vi "InitializeSlowDAQ.vi"(11 "Negative Channels in":i32[](array[numeric])=[3, 5, 7, 9, 199, 199, 199, 199, 199, 199, 199]) -> (0 "error out":errorcluster, 1 "Handle Out":i32, 2 "IO Types Out":string[](array[string]), 3 "Positive Channels 2":i32[](array[numeric])=[2, 4, 6, 8, 0, 1, 10, 11, 12, 13, 14], 5 "Negative Channels out":i32[](array[numeric])=[3, 5, 7, 9, 199, 199, 199, 199, 199, 199, 199])   [LabVIEW 2022 SP3]
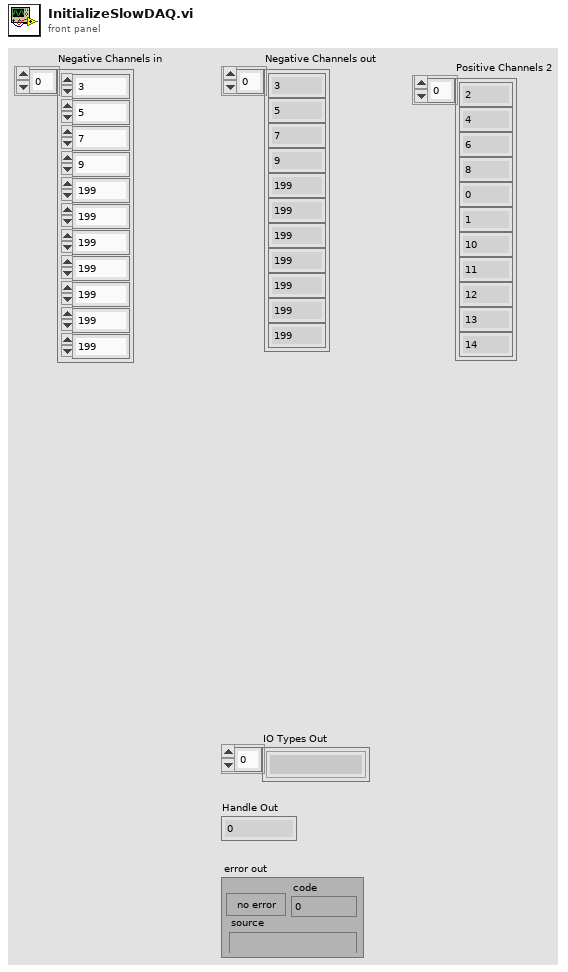
[diagram p1: front panel]
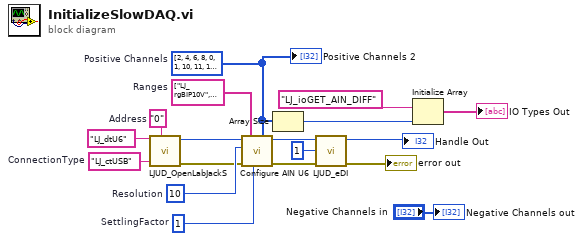
[diagram p0: block diagram]
diagram:
  w10 = string[] ["LJ_rgBIP10V", "LJ_rgBIP10V", "LJ_rgBIP10V", "LJ_rgBIP10V", "LJ_rgBIP1V", "LJ_rgBIP1V", "LJ_rgBIP1V", "LJ_rgBIP1V", "LJ_rgBIP1V", "LJ_rgBIP1V", "LJ_rgBIP10V"]  # Ranges
  w14 = i32[] [2, 4, 6, 8, 0, 1, 10, 11, 12, 13, 14]  # Positive Channels
  w7 = 1  # SettlingFactor
  w6 = 10  # Resolution
  w1 = "0"  # Address
  w3 = "LJ_ctUSB"  # ConnectionType
  n1 = call <vilib>:"LJUD_OpenLabJackS.vi"("Address"=w1, "ConnectionType"=w3, "DeviceType"="LJ_dtU6") -> ("error out"=w5:errorcluster, "Handle"=w4:i32)  [unwired: 6 in, 1 out]
  n2 = call <vilib>:"Configure AIN U6.vi"("Ranges"=w10, "SettlingFactor"=w7, "Positive Channels"=w14, "error in"=w5, "Resolution"=w6, "Handle In"=w4) -> ("error out"=w9:errorcluster, "Handle Out"=w8:i32)  [unwired: 4 in]
  n3 = Array Size(array=w14) -> (size(s)=w12:i32)
  n4 = call <vilib>:"LJUD_eDI.vi"("error in"=w9, "Channel"=1, "Handle In"=w8) -> ("error out"=→"error out":errorcluster, "Handle Out"=→"Handle Out":i32)  [unwired: 6 in, 1 out]
  n5 = Initialize Array("LJ_ioGET_AIN_DIFF" ("IOType"), w12) -> (→"IO Types Out":string[])
  "Positive Channels 2" <- w14
  "Negative Channels out" <- "Negative Channels in"
